vi "Mcp2210 Set Gpio Config.vi"(6 "error in (no error)":errorcluster, 7 "GPIO CFG":T2, 8 "Chip Setting Selection":T1(ring), 9 "handle":i32) -> (0 "error out":errorcluster, 3 "handle out":i32)   [LabVIEW 2015, in "mcp2210.lvlib"]
doc: "Set the current GPIO configuration or the power-up default (NVRAM) GPIO configuration.\nIf the chip NVRAM is password protected, the power-up GPIO configuration cannot be executed, the API\nreturns M_E_ERR_BLOCKED_ACCESS.\nParameters:\nInputs:\n- IntPtr handle - The pointer to the device handle. Cannot be NULL.\n- unsigned char cfgSelector - current/power-up chip setting selection. Valid values are:\n- M_MCP2210_VM_CONFIG: designates current chip setting (Volatile\nMemory)\n- M_MCP2210_NVRAM_CONFIG: designates power-up chip setting (NVRAM)\n- array<Byte> ^pGpioPinDes - GPIO Pin Designation array. Cannot be NULL.\nArray length is M_MCP2210_GPIO_NR\nValid values for pin designation are:\n- M_MCP2210_PIN_DES_GPIO\n- M_MCP2210_PIN_DES_CS\n- M_MCP2210_PIN_DES_FN\n- unsigned int dfltGpioOutput - GPIO pin output values.\n- unsigned int dfltGpioDir - GPIO pin direction.\n- unsigned char rmtWkupEn - remote wake-up setting. Valid values:\n- M_MCP2210_REMOTE_WAKEUP_ENABLED\n- M_MCP2210_REMOTE_WAKEUP_DISABLED\n- unsigned char intPinMd - interrupt pulse count mode. Valid values are:\n- M_MCP2210_INT_MD_CNT_HIGH_PULSES\n- M_MCP2210_INT_MD_CNT_LOW_PULSES\n- M_MCP2210_INT_MD_CNT_RISING_EDGES\n- M_MCP2210_INT_MD_CNT_FALLING_EDGES\n- M_MCP2210_INT_MD_CNT_NONE\n- unsigned char spiBusRelEn - SPI Bus Release option. Valid values are:\n- M_MCP2210_SPI_BUS_RELEASE_ENABLED\n- M_MCP2210_SPI_BUS_RELEASE_DISABLED\nOutputs:\n- none\nReturns:\n- 0 for success: M_E_SUCCESS\n- negative error code: M_E_ERR_NULL, M_E_ERR_INVALID_HANDLE_VALUE\nM_E_ERR_UNKOWN_ERROR, M_E_ERR_INVALID_PARAMETER\nM_E_ERR_HID_TIMEOUT, M_E_ERR_HID_RW_FILEIO\nM_E_ERR_BLOCKED_ACCESS\nM_E_ERR_CMD_ECHO, M_E_ERR_CMD_FAILED\n\nMCP2210_DLL_UM_API int __stdcall Mcp2210_SetGpioConfig(void *handle, unsigned char cfgSelector, unsigned char *pGpioPinDes, unsigned int dfltGpioOutput,\n unsigned int dfltGpioDir, unsigned char rmtWkupEn, unsigned char intPinMd, unsigned char spiBusRelEn);"
uses:
  <userlib>/mcp2210/mcp2210.lvlib
  <userlib>/mcp2210/mcp2210_dll_um_x86.dll
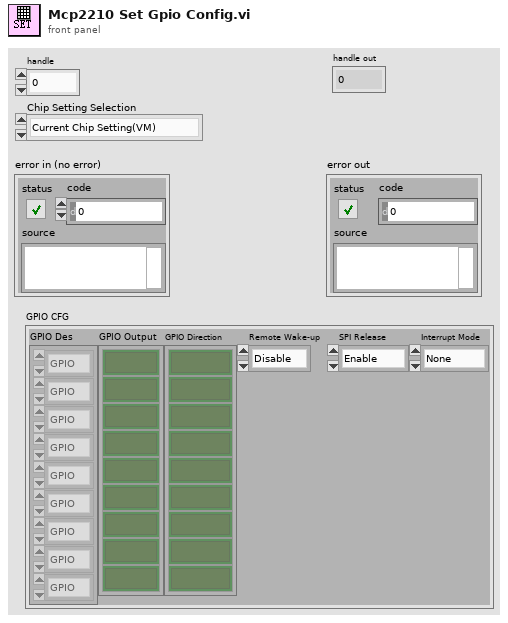
[diagram p1: front panel]
types:
  T1 = enum8{"Current Chip Setting(VM)", "Power-up Chip Setting(NVRAM)"}
  T2 = cluster{"GPIO Des":enum8{"GPIO", "CS", "Dedicated"}[], "GPIO Output":bool[], "GPIO Direction":bool[], "Remote Wake-up":enum8{"Disable", "Enable"}, "SPI Release":enum16{"Enable", "Disable"}, "Interrupt Mode":enum8{"None", "Falling", "Rising", "Low", "High"}}
  T3 = enum8{"None", "Falling", "Rising", "Low", "High"}
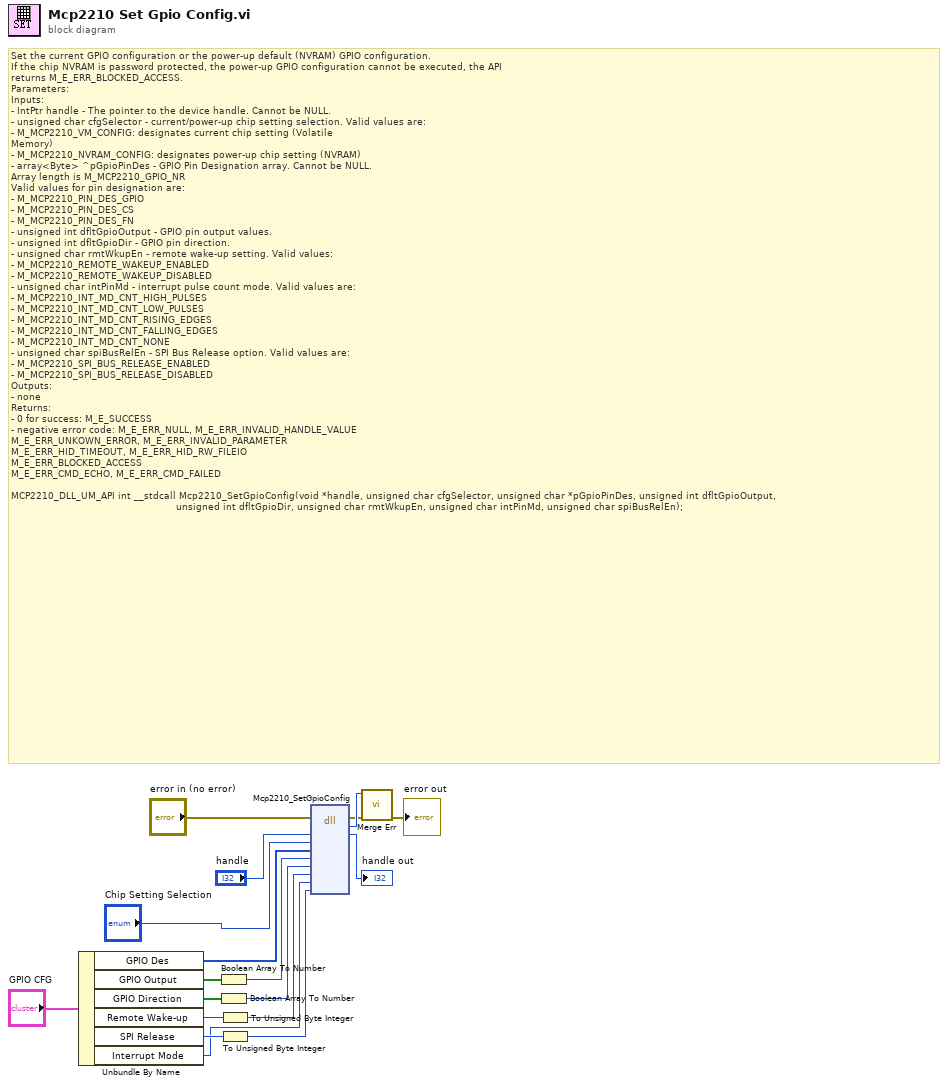
[diagram p0: block diagram]
diagram:
  # "Set the current GPIO configuration or the power-up default (NVRAM) GPIO configuration.\nIf the chip NVRAM is password protected, the power-up GPIO configuration cannot be executed, the API\nreturns M_E_ERR_BLOCKED_ACCESS.\nParameters:\nInputs:\n- IntPtr handle - The pointer to the device handle. Cannot be NULL.\n- unsigned char cfgSelector - current/power-up chip setting selection. Valid values are:\n- M_MCP2210_VM_CONFIG: designates current chip setting (Volatile\nMemory)\n- M_MCP2210_NVRAM_CONFIG: designates power-up chip setting (NVRAM)\n- array<Byte> ^pGpioPinDes - GPIO Pin Designation array. Cannot be NULL.\nArray length is M_MCP2210_GPIO_NR\nValid values for pin designation are:\n- M_MCP2210_PIN_DES_GPIO\n- M_MCP2210_PIN_DES_CS\n- M_MCP2210_PIN_DES_FN\n- unsigned int dfltGpioOutput - GPIO pin output values.\n- unsigned int dfltGpioDir - GPIO pin direction.\n- unsigned char rmtWkupEn - remote wake-up setting. Valid values:\n- M_MCP2210_REMOTE_WAKEUP_ENABLED\n- M_MCP2210_REMOTE_WAKEUP_DISABLED\n- unsigned char intPinMd - interrupt pulse count mode. Valid values are:\n- M_MCP2210_INT_MD_CNT_HIGH_PULSES\n- M_MCP2210_INT_MD_CNT_LOW_PULSES\n- M_MCP2210_INT_MD_CNT_RISING_EDGES\n- M_MCP2210_INT_MD_CNT_FALLING_EDGES\n- M_MCP2210_INT_MD_CNT_NONE\n- unsigned char spiBusRelEn - SPI Bus Release option. Valid values are:\n- M_MCP2210_SPI_BUS_RELEASE_ENABLED\n- M_MCP2210_SPI_BUS_RELEASE_DISABLED\nOutputs:\n- none\nReturns:\n- 0 for success: M_E_SUCCESS\n- negative error code: M_E_ERR_NULL, M_E_ERR_INVALID_HANDLE_VALUE\nM_E_ERR_UNKOWN_ERROR, M_E_ERR_INVALID_PARAMETER\nM_E_ERR_HID_TIMEOUT, M_E_ERR_HID_RW_FILEIO\nM_E_ERR_BLOCKED_ACCESS\nM_E_ERR_CMD_ECHO, M_E_ERR_CMD_FAILED\n\nMCP2210_DLL_UM_API int __stdcall Mcp2210_SetGpioConfig(void *handle, unsigned char cfgSelector, unsigned char *pGpioPinDes, unsigned int dfltGpioOutput,\n                                                       unsigned int dfltGpioDir, unsigned char rmtWkupEn, unsigned char intPinMd, unsigned char spiBusRelEn);"
  n1 = Unbundle By Name("GPIO CFG") -> ("GPIO Des"=w15:enum8{"GPIO", "CS", "Dedicated"}[], "GPIO Output"=w10:bool[], "GPIO Direction"=w8:bool[], "Remote Wake-up"=w6:enum8{"Disable", "Enable"}, "SPI Release"=w4:enum16{"Enable", "Disable"}, "Interrupt Mode"=w2:T3)
  n2 = Boolean Array To Number(Boolean array=w10) -> (number=w9:u32)
  n3 = Boolean Array To Number(Boolean array=w8) -> (number=w7:u32)
  n4 = To Unsigned Byte Integer(number=w6) -> (unsigned 8bit integer=w5:u8)
  n5 = To Unsigned Byte Integer(number=w4) -> (unsigned 8bit integer=w3:u8)
  n6 = dll-call lib="D:/LabVIEW 2015/user.lib/mcp2210/mcp2210_dll_um_x86.*" fn="Mcp2210_SetGpioConfig"(error in="error in (no error)", "handle"="handle", "cfgSelector"="Chip Setting Selection", "pGpioPinDes"=w15, "dfltGpioOutput"=w9, "dfltGpioDir"=w7, "rmtWkupEn"=w5, "intPinMd"=w2, "spiBusRelEn"=w3) -> (error out=w13:errorcluster, "return type"=w14:i32, "handle"=→"handle out":i32)  [unwired: 9 in, 1 out]
  n7 = call <userlib>:"Merge Err.vi"("error in (no error)"=w13, "return type"=w14) -> ("error out"=→"error out":errorcluster)  [unwired: 9 in]
